vi "MEE5318_Project1_DuffyWalker.vi"() -> ()   [LabVIEW 2021]
uses:
  <vilib>/Analysis/3filter.llb/Filter Structure Type.ctl
  <vilib>/DAQmx/read.llb/DAQmx Read (Counter DBL 1Chan 1Samp).vi
  <vilib>/DAQmx/read.llb/DAQmx Read (Analog 1D Wfm NChan 1Samp).vi
  <vilib>/DAQmx/create/channels.llb/DAQmx Create Channel (AI-Voltage-Basic).vi
  <vilib>/DAQmx/create/channels.llb/DAQmx Create Channel (CI-Position-Angular Encoder).vi
  <vilib>/DAQmx/configure/timing.llb/DAQmx Timing (Sample Clock).vi
  <vilib>/Utility/file.llb/Write Delimited Spreadsheet (string).vi
  <vilib>/DAQmx/miscellaneous.llb/DAQmx Fill In Error Info.vi
  <vilib>/measure/macond.llb/IIR Filter for 1 Chan.vi
  <vilib>/Waveform/WDTOps.llb/WDT Get Waveform Time Array DBL.vi
  <vilib>/Utility/file.llb/Write Delimited Spreadsheet (DBL).vi
  <vilib>/measure/NI_MAPro.lvlib
  <resource>/objmgr/daqmx.rc
  <vilib>/Analysis/NI_AALBase.lvlib
panel:
  in  "Digital Filter Specs":T1={"Topology"=enum."Butterworth", "Type"=enum."Lowpass", "Order"=1, "Lower Fc"=100.0, "Upper Fc"=200.0, "PB Ripple"=1.0, "SB Attenuation"=60.0} {"PB Ripple" format="%0.2f"; "SB Attenuation" format="%0.2f"; "Lower Fc" format="%0.2p"; "Upper Fc" format="%0.2p"}
  in  "Max Samples":i32=1000
  out "Encoder Position":waveform(dbl)[](graph)
  in  "Pulses Per Revolution":u32=24
  in  "B Input Terminal":tag="PFI10"
  in  "A Input Terminal":tag="PFI8"
  in  "Counter":tag="Dev1/ctr0"
  in  "Path":path
  in  "Calibration Constant":dbl
  in  "Sample Rate (hz)":dbl=1000.0 format="%0.2f"
  in  "Analog Filter Specs":T1={"Topology"=enum."Butterworth", "Type"=enum."Lowpass", "Order"=1, "Lower Fc"=100.0, "Upper Fc"=200.0, "PB Ripple"=1.0, "SB Attenuation"=60.0} {"PB Ripple" format="%0.2f"; "SB Attenuation" format="%0.2f"; "Lower Fc" format="%0.2p"; "Upper Fc" format="%0.2p"}
  out "Analog Input 1":waveform(dbl)[](graph)
  in  "Analog Channels":tag
  in  "stop":bool
  out "Analog Input 0":waveform(dbl)[](graph)
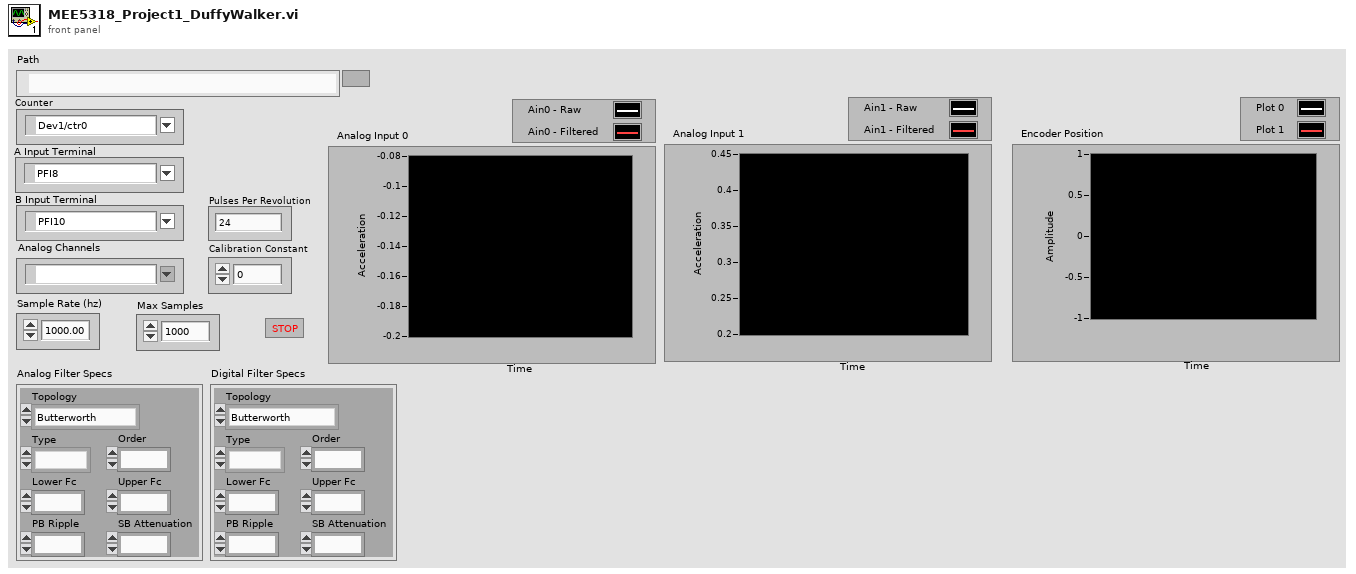
[diagram p1: front panel]
types:
  T1 = cluster{"Topology":enum16{"Off", "Butterworth", "Chebyshev", "Inverse Chebyshev", "Elliptic", "Bessel"}, "Type":enum16{"Lowpass", "Highpass", "Bandpass", "Bandstop"}, "Order":i32, "Lower Fc":dbl, "Upper Fc":dbl, "PB Ripple":dbl, "SB Attenuation":dbl}
  T2 = typedef "NI_AALBase.lvlib/Filter Structure Type.ctl" = u16
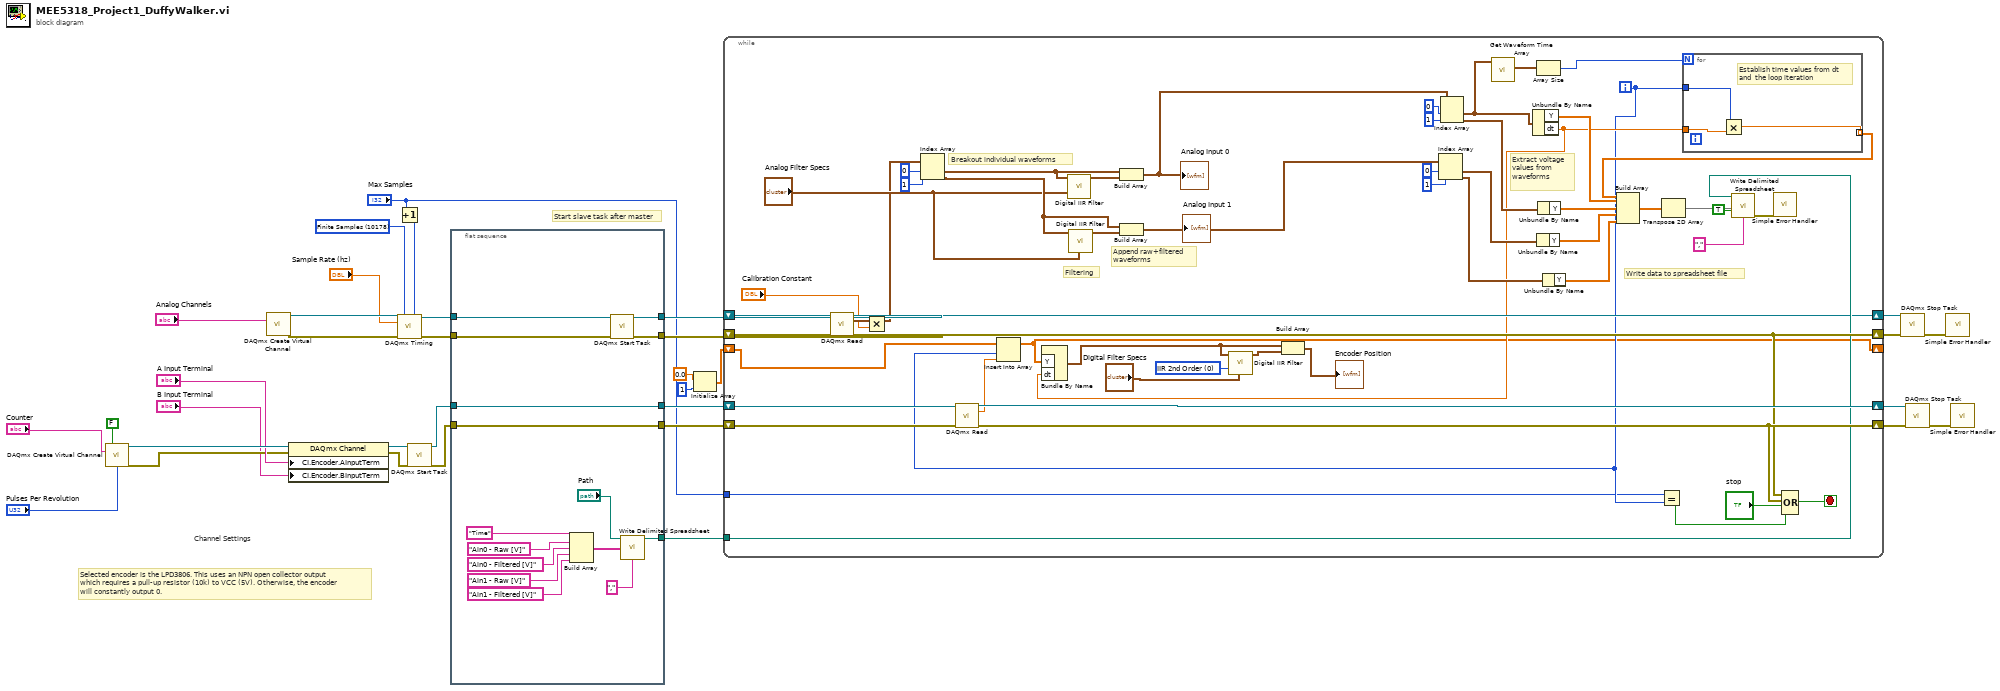
[diagram p0: block diagram]
diagram:
  w16 = 10178 items=["Finite Samples"=10178, "Continuous Samples"=10123, "Hardware Timed Single Point"=12522] ("sample mode")
  # "Channel Settings"
  # "Start slave task after master"
  # "Selected encoder is the LPD3806. This uses an NPN open collector output\nwhich requires a pull-up resistor (10k) to VCC (5V). Otherwise, the encoder\nwill constantly output 0."
  n1 = call-poly <vilib>:"DAQmx Create Virtual Channel.vi"("z index enable"=FALSE, "counter"="Counter", "pulses per revolution"="Pulses Per Revolution") -> ("task out"=w13:refnum<k21>, "error out"=w11:errorcluster)  [unwired: 11 in]
  n2 = call-poly <vilib>:"DAQmx Create Virtual Channel.vi"("physical channels"="Analog Channels") -> ("task out"=w21:refnum<k21>, "error out"=w19:errorcluster)  [unwired: 13 in]
  n3 = property class="DAQmx Channel"(reference=w13, error in=w11, "CI.Encoder.AInputTerm"="A Input Terminal", "CI.Encoder.BInputTerm"="B Input Terminal") -> (reference out=w8:refnum<k21>, error out=w7:errorcluster)
  n4 = Increment(x="Max Samples") -> (x+1=w1:i32)
  n5 = call-poly <vilib>:"DAQmx Timing.vi"("task/channels in"=w21, "sample mode"=w16, "samples per channel"=w1, "rate"="Sample Rate (hz)", "error in"=w19) -> ("task out"=w20:refnum<k21>, "error out"=w18:errorcluster)  [unwired: 9 in]
  n6 = call <vilib>:"DAQmx Start Task.vi"("task/channels in"=w8, "error in"=w7) -> ("task out"=w25:refnum<k21>, "error out"=w23:errorcluster)  [unwired: 12 in]
  n7 = flat-sequence {
    tunnel: [w49] -> w34
    tunnel: [w48] -> w33
    tunnel: w20 -> [w47]
    tunnel: w18 -> [w46]
    tunnel: w25 -> [w45]
    tunnel: [w45] -> w24
    tunnel: w23 -> [w44]
    tunnel: [w44] -> w22
    tunnel: [w41] -> w15
    frame #0 {
      n8 = Build Array("Time", "Ain0 - Raw [V]", "Ain0 - Filtered [V]", "Ain1 - Raw [V]", "Ain1 - Filtered [V]") -> (w35:string[])
      n9 = call <vilib>:"DAQmx Start Task.vi"("task/channels in"=w47, "error in"=w46) -> ("task out"=w48:refnum<k21>, "error out"=w49:errorcluster)  [unwired: 12 in]
      n10 = call-poly <vilib>:"Write Delimited Spreadsheet.vi"("file path (dialog if empty)"="Path", "1D data"=w35, "delimiter (\\t)"="," ("delimiter (\\t)")) -> ("new file path (Not A Path if cancelled)"=w41:path)  [unwired: 11 in, 1 out]
    }
  }
  n11 = Initialize Array(0.0 ("element"), 1 ("dimension size")) -> (w3:dbl[])
  n12 = while {
    shift-right: [w101] -> w31
    shift-left: w34 -> [w95]
    shift-right: [w62] -> w32
    shift-left: w33 -> [w96]
    shift-right: [w103] -> w28
    shift-left: w24 -> [w94]
    shift-right: [w102] -> w27
    shift-left: w22 -> [w93]
    tunnel: w15 -> [w63]
    shift-right: [w51] -> _
    shift-left: w3 -> [w54]
    tunnel: "Max Samples" -> [w50]
    i -> [w52]
    stop <- w104 stop-if-true
    w56 = T2 0 items=["IIR 2nd Order"=0, "IIR 4th Order"=1, "Auto Select"=10] ("filter structure option")
    # "Extract voltage values from waveforms"
    # "Write data to spreadsheet file"
    # "Breakout individual waveforms"
    # "Append raw+filtered\nwaveforms"
    # "Filtering"
    n13 = call-poly <vilib>:"DAQmx Read.vi"("task/channels in"=w96, "error in"=w95) -> ("task out"=w62:refnum<k21>, "data"=w99:waveform(dbl)[], "error out"=w101:errorcluster)  [unwired: 11 in]
    n14 = Multiply(x=w99, y="Calibration Constant") -> (x*y=w87:waveform(dbl)[])
    n15 = Index Array(array=w87, index #1=0 ("index"), index #2=1 ("index")) -> (element #1=w88:waveform(dbl), element #2=w90:waveform(dbl))
    n16 = call-poly <vilib>:"DAQmx Read.vi"("task/channels in"=w94, "error in"=w93) -> ("task out"=w103:refnum<k21>, "data"=w53:dbl, "error out"=w102:errorcluster)  [unwired: 11 in]
    n17 = Insert Into Array(array=w54, index=w52, new element=w53) -> (w51:dbl[])
    n18 = call-poly <vilib>:"Digital IIR Filter.vi"("IIR filter specifications"="Analog Filter Specs", "signal in"=w88) -> ("signal out"=w92:waveform(dbl))  [unwired: 7 in, 2 out]
    n19 = call-poly <vilib>:"Digital IIR Filter.vi"("IIR filter specifications"="Analog Filter Specs", "signal in"=w90) -> ("signal out"=w91:waveform(dbl))  [unwired: 7 in, 2 out]
    n20 = Build Array(w88, w92) -> (w85:waveform(dbl)[])
    "Analog Input 0" <- w85
    n21 = Build Array(w90, w91) -> (w84:waveform(dbl)[])
    "Analog Input 1" <- w84
    n22 = Index Array(array=w84, index #1=0 ("index"), index #2=1 ("index")) -> (element #1=w76:waveform(dbl), element #2=w77:waveform(dbl))
    n23 = Index Array(array=w85, index #1=0 ("index"), index #2=1 ("index")) -> (element #1=w74:waveform(dbl), element #2=w75:waveform(dbl))
    n24 = call-poly <vilib>:"Get Waveform Time Array.vi"("waveform in"=w74) -> ("X array"=w73:timestamp[])  [unwired: 9 in, 1 out]
    n25 = Unbundle By Name(w74) -> ("Y"=w80:dbl[], "dt"=w61:dbl)
    n26 = Bundle By Name("Y"=w51, "dt"=w61) -> (w55:waveform(dbl))  [unwired: 1 in]
    n27 = call-poly <vilib>:"Digital IIR Filter.vi"("IIR filter specifications"="Digital Filter Specs", "filter structure option"=w56, "signal in"=w55) -> ("signal out"=w58:waveform(dbl))  [unwired: 6 in, 2 out]
    n28 = Build Array(w55, w58) -> (→"Encoder Position":waveform(dbl)[])
    n29 = Array Size(array=w73) -> (size(s)=w72:i32)
    n30 = Unbundle By Name(w76) -> ("Y"=w82:dbl[])
    n31 = Unbundle By Name(w75) -> ("Y"=w81:dbl[])
    n32 = Unbundle By Name(w77) -> ("Y"=w83:dbl[])
    n33 = Equal?(x=w50, y=w52) -> (x = y?=w60:bool)
    n34 = for {
      N: w72 -> [_]
      tunnel: w61 -> [w106]
      tunnel: [w105] -> w79 mode=indexing
      tunnel: w52 -> [w107]
      # "Establish time values from dt\nand  the loop iteration"
      n35 = Multiply(x=w107, y=w106) -> (x*y=w105:dbl)
    }
    n36 = Build Array(w79, w80, w81, w82, w83) -> (w78:dbl[][])
    n37 = Transpose 2D Array(2D array=w78) -> (transposed array=w66:dbl[][])
    n38 = call-poly <vilib>:"Write Delimited Spreadsheet.vi"("file path (dialog if empty)"=w63, "2D data"=w66, "append to file? (new file:F)"=TRUE, "delimiter (\\t)"=",") -> ("error out"=w64:errorcluster)  [unwired: 10 in, 1 out]
    n39 = call <vilib>:"Simple Error Handler.vi"("error in (no error)"=w64) -> ()  [unwired: 4 in, 5 out]
    n40 = Compound Arithmetic op=OR(w101, w102, "stop", w60) -> (w104:bool)
  }
  n41 = call <vilib>:"DAQmx Stop Task.vi"("task/channels in"=w32, "error in"=w31) -> ("error out"=w30:errorcluster)  [unwired: 12 in, 1 out]
  n42 = call <vilib>:"DAQmx Stop Task.vi"("task/channels in"=w28, "error in"=w27) -> ("error out"=w29:errorcluster)  [unwired: 12 in, 1 out]
  n43 = call <vilib>:"Simple Error Handler.vi"("error in (no error)"=w30) -> ()  [unwired: 4 in, 5 out]
  n44 = call <vilib>:"Simple Error Handler.vi"("error in (no error)"=w29) -> ()  [unwired: 4 in, 5 out]
